vi "As PropertyObject.vi"(8 "error in (no error)":errorcluster, 11 "UIMessage in":refnum<class "UIMessage.lvclass">) -> (0 "error out":errorcluster, 2 "PropertyObject":refnum<k7>, 3 "UIMessage out":refnum<class "UIMessage.lvclass">)   [LabVIEW 2020, in "TSnax.lvlib" / "UIMessage.lvclass"]
uses:
  UIMessage.lvclass
  UIMessage.lvclass/UIMessage.ctl
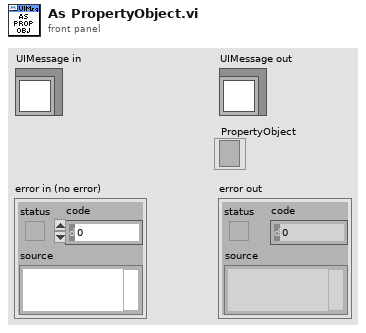
[diagram p1: front panel]
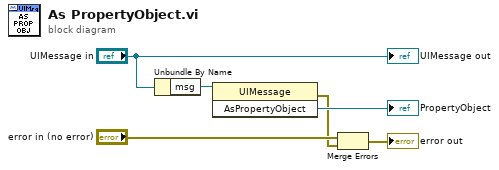
[diagram p0: block diagram]
diagram:
  n1 = Unbundle By Name("UIMessage in") -> ("msg"=w4:refnum<k7>)
  n2 = invoke class="UIMessage" method="AsPropertyObject"(reference=w4) -> (error out=w1:errorcluster, "AsPropertyObject"=→"PropertyObject":refnum<k7>)  [unwired: 2 in, 1 out]
  n3 = Merge Errors("error in (no error)", w1) -> (→"error out":errorcluster)
  "UIMessage out" <- "UIMessage in"
